vi "Snap SN.vi"(11 "Main Page UIRef":T1) -> (0 "error out":errorcluster)   [LabVIEW 2019, in "MPC_Laser Marked.lvclass"]
uses:
  MPC_Laser Marked.lvclass
  Function/IO Folder/IO_VI/IOCtrl/Ctrl/DMC1000B_1 SelectOutput.ctl
  Function/UpVision/Ctrl/UpGrayImg.ctl
  Function/UpVision/Ctrl/UpColorImg.ctl
  Function/UpVision/Ctrl/UpEnum_VisionCalibSet_Act.ctl
  Function/Main UI/Glb/Main_UI Gb.vi
  LLB/Message/MsgShowAndLog.lvlib
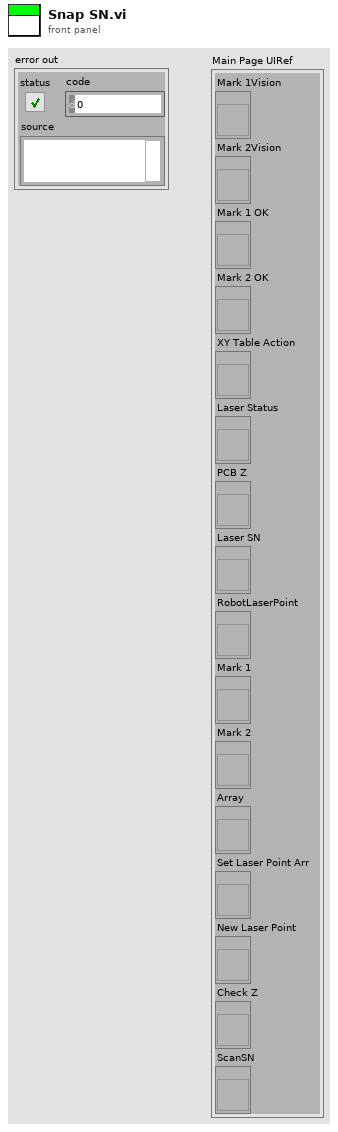
[diagram p1: front panel]
types:
  T1 = cluster{"Mark 1Vision":refnum<vi>, "Mark 2Vision":refnum<vi>, "Mark 1 OK":refnum<vi>, "Mark 2 OK":refnum<vi>, "XY Table Action":refnum<vi>, "Laser Status":refnum<vi>, "PCB Z":refnum<vi>, "Laser SN":refnum<vi>, "RobotLaserPoint":refnum<vi>, "Mark 1":refnum<vi>, "Mark 2":refnum<vi>, "Array":refnum<vi>, "Set Laser Point Arr":refnum<vi>, "New Laser Point":refnum<vi>, "Check Z":refnum<vi>, "ScanSN":refnum<vi>}
  T2 = typedef "UpGrayImg.ctl" = enum16{"CUpGray", "CUpProce1", "CUpProce2", "UpPattern1", "UpPattern2", "UpCalibImg", "UpPreProcess"}
  T3 = typedef "UpColorImg.ctl" = enum16{"CUpCam", "CUpSource", "CUpShow", "CUpToProcess1", "CUpToProcess2", "CUpForMatch", "CUpForCheckNumbers", "CupPreProcess"}
  T4 = typedef "DMC1000B_1 SelectOutput.ctl" = enum16{"M_Out0預備", "M_OUT01蜂鳴器", "M_OUT02紅燈", "M_OUT03綠燈", "M_OUT04黃燈", "M_OUT05上頂固定位氣缸電磁閥", "M_OUT06到料阻擋氣缸電磁閥", "M_OUT07向前機台發出要料#1信號", "M_OUT08向前機台發出要料#2信號", "M_OUT09向後機台發出有料#3信號", "M_OUT10向後機台發出有料#4信號", "M_OUT11接駁台馬達啟動開/關", "M_OUT12接駁台馬達慢速", "M_OUT13抽風機開/關", "M_OUT14上視覺上光源", "M_OUT15DC吹風扇開/關", "M_OUT16Z軸煞車釋放", "M_OUT17", "M_OUT18", "M_OUT19", "M_OUT20", "M_OUT21", "M_OUT22", "M_OUT23", "M_OUT24", "M_OUT25第一軸SEVON1伺服使能信號", "M_OUT26第二軸SEVON2伺服使能信號", "M_OUT27第三軸SEVON3伺服使能信號"}
  T5 = typedef "UpEnum_VisionCalibSet_Act.ctl" = enum16{"initial", "initialref", "save", "load", "UpDataToUI", "write", "read"}
  T6 = typedef "IMAQ Image.ctl" = refnum<image>
  T7 = typedef "QR Code Report.ctl" = cluster{"Found?":bool, "Data":string, "Bounding Box":cluster{"x":sgl, "y":sgl}[], "Errors Corrected":u32, "Dimensions (Rows/Cols)":u32, "Version":u32, "QR Model":T8, "Stream Mode":T9, "Barcode Polarity":T10, "Mirrored?":bool, "Append Stream Position":u32, "Size of Append Stream":u32, "First EAN-128 ID":i32, "First Alternate Language ID":i32, "Append Stream ID":u32, "Minimum Edge Strength":u32, "Demodulation Mode":T11, "Cell Sample Size":T12, "Cell Filter Mode":T13}
  T8 = typedef "QR Code Model Type.ctl" = i32
  T9 = typedef "QR Code Stream Mode Type.ctl" = i32
  T10 = typedef "Data Matrix Polarity.ctl" = i32
  T11 = typedef "Demodulation Mode.ctl" = i32
  T12 = typedef "Cell Sample Size.ctl" = i32
  T13 = typedef "Cell Filter Mode.ctl" = i32
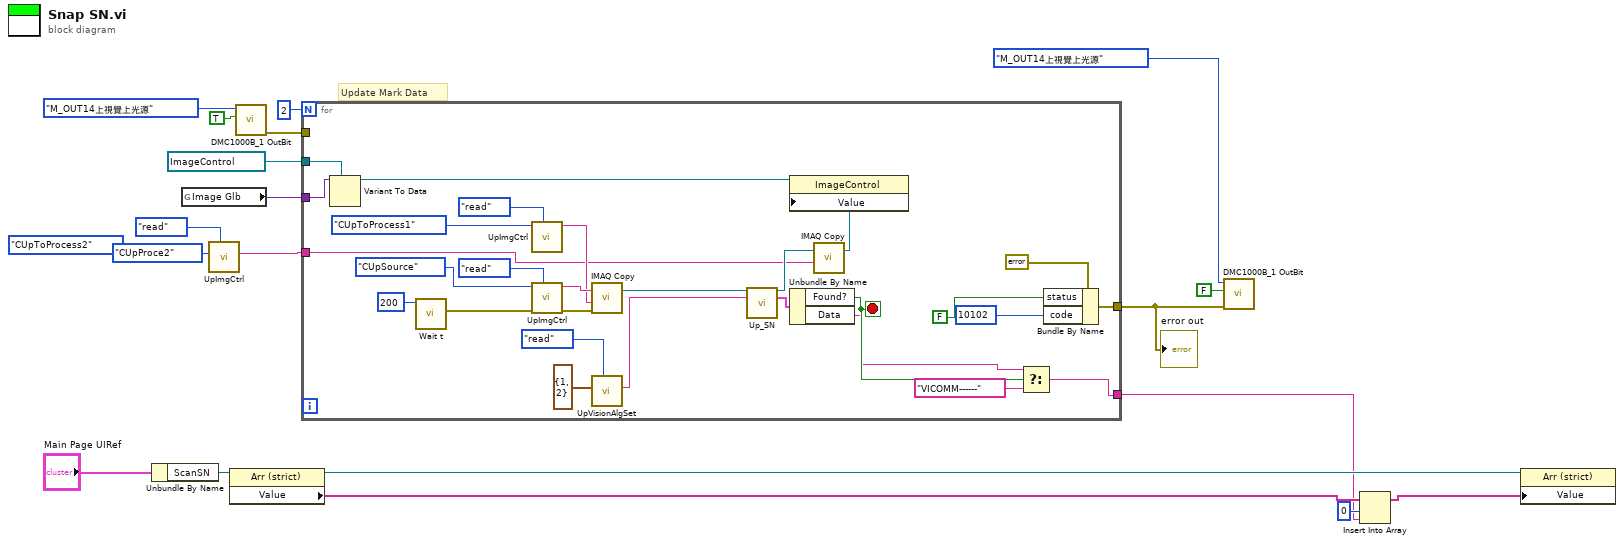
[diagram p0: block diagram]
diagram:
  (unwired) UpColorImg."CUpToProcess2" ("ColorImg 2")
  # "Update Mark Data"
  n1 = Unbundle By Name("Main Page UIRef") -> ("ScanSN"=w9:refnum<vi>)
  n2 = global read "Main_UI Gb.vi" "Image Glb"() -> (w18:variant)
  n3 = call "UpImgCtrl.vi"("Action"=enum16{"Initial", "read", "release"}."read", "GrayImg 2"=UpGrayImg."CUpProce2") -> ("GrayImg"=w2:string)  [unwired: 7 in, 2 out]
  n4 = property class="Arr (strict)"(reference=w9) -> (reference out=w7:refnum<vi>, "Value"=w8:string[])  [unwired: 1 in, 1 out]
  n5 = call "DMC1000B_1 OutBit.vi"("BL"=TRUE, "IO_Output_1 Select"=DMC1000B_1_SelectOutput."M_OUT14上視覺上光源") -> ("error out"=w14:errorcluster)  [unwired: 9 in]
  n6 = for {
    N: 2 -> [_]
    tunnel: [w36] -> w17
    tunnel: w14 -> [_]
    tunnel: w18 -> [w33]
    tunnel: refnum<vi> refnum ("Image") -> [w32]
    tunnel: [w24] -> w4
    tunnel: w2 -> [w21]
    stop <- w26 stop-if-true
    n7 = Variant To Data(type=w32, Variant=w33) -> (data=w31:refnum<vi>)  [unwired: 1 in, 1 out]
    n8 = call "Wait t.vi"("wait(ms)"=u32 200) -> ("error out"=w40:errorcluster)  [unwired: 10 in]
    n9 = call "UpImgCtrl.vi"("Action"=enum16{"Initial", "read", "release"}."read", "ColorImg 2"=UpColorImg."CUpToProcess1") -> ("ColorImg"=w41:string)  [unwired: 7 in, 2 out]
    n10 = call "UpImgCtrl.vi"("Action"=enum16{"Initial", "read", "release"}."read", "error in (no error)"=w40, "ColorImg 2"=UpColorImg."CUpSource") -> ("error out"=w39:errorcluster, "ColorImg"=w42:string)  [unwired: 6 in, 1 out]
    n11 = call "IMAQ Copy"("error in (no error)"=w39, "Image Dst"=w41, "Image Src"=w42) -> ("Image Dst Out"=w30:T6)  [unwired: 3 in, 1 out]
    n12 = call "UpVisionAlgSet.vi"("Enum"=UpEnum_VisionCalibSet_Act."read", "indedx"=cluster{"Y":i32, "X":i32} {"Y"=1, "X"=2}) -> ("DataOut"=w29:string)  [unwired: 7 in, 2 out]
    n13 = call "Up_SN.vi"("Image Src"=w30, "ROIIn"=w29) -> ("Image Out"=w22:T6, "QR Code Report"=w28:T7)  [unwired: 11 in, 1 out]
    n14 = Unbundle By Name(w28) -> ("Found?"=w26:bool, "Data"=w25:string)
    n15 = call "IMAQ Copy"("Image Dst"=w21, "Image Src"=w22) -> ("Image Dst Out"=w20:T6)  [unwired: 4 in, 1 out]
    n16 = property class="ImageControl"(reference=w31, "Value"=w20) -> ()  [unwired: 1 in, 2 out]
    n17 = Select(t=w25, s=w26, f="VICOMM------") -> (s? t:f=w24:string)
    n18 = Bundle By Name(cluster=errorcluster {"status"=FALSE, "code"=0, "source"=""} ("error constant"), "status"=FALSE, "code"=10102) -> (w36:errorcluster)
  }
  "error out" <- w17
  n19 = call "DMC1000B_1 OutBit.vi"("error in (no error)"=w17, "BL"=FALSE, "IO_Output_1 Select"=DMC1000B_1_SelectOutput."M_OUT14上視覺上光源") -> ()  [unwired: 8 in, 1 out]
  n20 = Insert Into Array(array=w8, index=0, new element=w4) -> (w6:string[])
  n21 = property class="Arr (strict)"(reference=w7, "Value"=w6) -> ()  [unwired: 1 in, 2 out]
